vi "MotionProfiles_Control.vi"(8 "error in (no error)":errorcluster, 11 "MotionProfiles in":refnum<class "MotionProfiles.lvclass">) -> (0 "error out":errorcluster, 3 "MotionProfiles out":refnum<class "MotionProfiles.lvclass">)   [LabVIEW 2016, in "MotionProfiles.lvclass"]
uses:
  MotionProfiles.lvclass
  MotionProfiles.lvclass/MotionProfiles.ctl
  MotionProfile_InternalStateEnum.ctl
  MotionProfile_TalonSetValueEnum.ctl
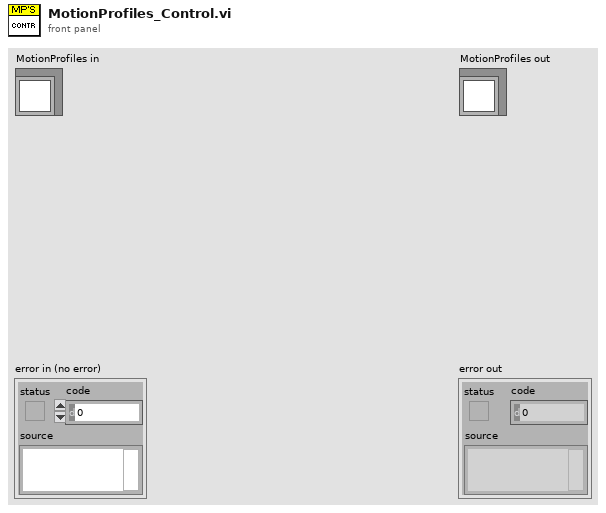
[diagram p1: front panel]
types:
  T1 = typedef "MotionProfiles.lvclass/MotionProfile_InternalStateEnum.ctl" = enum16{"Nothing", "Send Points to Talon", "Run Profile"}
  T2 = typedef "MotionProfiles.lvclass/MotionProfile_TalonSetValueEnum.ctl" = enum16{"Disable", "Enable", "Hold"}
  T3 = typedef "WPI_MotorControlDeviceRef.ctl" = cluster{"DeviceStatus":errorcluster, "Type":T4, "PWM":cluster{"PWM Channel":T5, "DeadBand":T6}, "CAN":cluster{"Device Number":u8, "SetOutput VI Ref":variant, "GetOutput VI Ref":variant, "Enable VI Ref":variant, "Disable VI Ref":variant, "Data":variant}, "Invert":bool}
  T4 = typedef "WPI_MotorControlType.ctl" = enum16{"PWM", "CAN"}
  T5 = typedef "FPGA_DIOPWMChannel.ctl" = enum8{"PWM 0", "PWM 1", "PWM 2", "PWM 3", "PWM 4", "PWM 5", "PWM 6", "PWM 7", "PWM 8", "PWM 9", "PWM MXP 0", "PWM MXP 1", "PWM MXP 2", "PWM MXP 3", "PWM MXP 4", "PWM MXP 5", "PWM MXP 6", "PWM MXP 7", "PWM MXP 8", "PWM MXP 9", "Invalid"}
  T6 = typedef "WPI_PWMDeadband.ctl" = cluster{"Name":string, "maxPositivePwm":i32, "minPositivePwm":i32, "centerPwm":i32, "maxNegativePwm":i32, "minNegativePwm":i32, "angularRange":u16}
  T7 = typedef "WPI_CANTalonSRX_GlobalStatus.ctl" = cluster{"Applied Throttle":dbl, "Module Enabled":bool, "CAN Error":errorcluster, "Closed Loop Error":dbl, "Forward Limit Switch Closed":bool, "Reverse Limit Switch Closed":bool, "Sensor Position":dbl, "Sensor Velocity":dbl, "Current":dbl, "Sticky Fault - Over Temp":bool, "Sticky Fault - Under Voltage":bool, "Sticky Fault - Forward Limit":bool, "Sticky Fault - Reverse Limit":bool, "Sticky Fault - Forward Soft Limit":bool, "Sticky Fault - Reverse Soft Limit":bool, "Brake is Enabled":bool, "Encoder Position":dbl, "Encoder Velocity":dbl, "Encoder Index Count":dbl, "Encoder A Pin State":bool, "Encoder B Pin State":bool, "Encoder Index Pin State":bool, "Analog In":dbl, "Analog In Velocity":dbl, "Temperature (C)":dbl, "Battery Voltage":dbl, "Control 5 Is Supported":bool, "Current Profile Slot Select":dbl, "Pos Div 8":bool, "Vel Div 4":bool, "Pulse Width Position":i32, "Pulse Width Velocity":i32, "Pulse Width Rise To Rise (us)":i32, "Pulse Width Rise To Fall (us)":i32, "Mot Prof Active Is Under Run":bool, "Mot Prof Active Has Under Run":bool, "Mot Prof Active Is Last":bool, "Mot Prof Active Velocity Only":bool, "Mot Prof Active Is Valid":bool, "Mot Prof Buffer Is Full":bool, "Mot Prof Active Profile Slot Select":i32, "Mot Prof NextID":i32, "Mot Prof Count":i32, "Mot Prof Active Velocity":dbl, "Mot Prof Active Position":dbl, "Mot Prof Output Enable":i32, "UsageFrame":u32, "Motion Magic Active Trajectory":cluster{"Velocity":dbl, "Position":dbl}}
  T8 = typedef "WPI_CANTalonSRX_MotionProfileTrajectoryPt.ctl" = cluster{"Duration Ms":u8, "Velocity":dbl, "Position":dbl, "Profile Slot Select":u8, "Is Last":bool, "Velocity Only":bool, "Zero Position":bool, "Compress Code":u8, "Same Velocity":i32, "Delta Position":i32, "Count":u8}
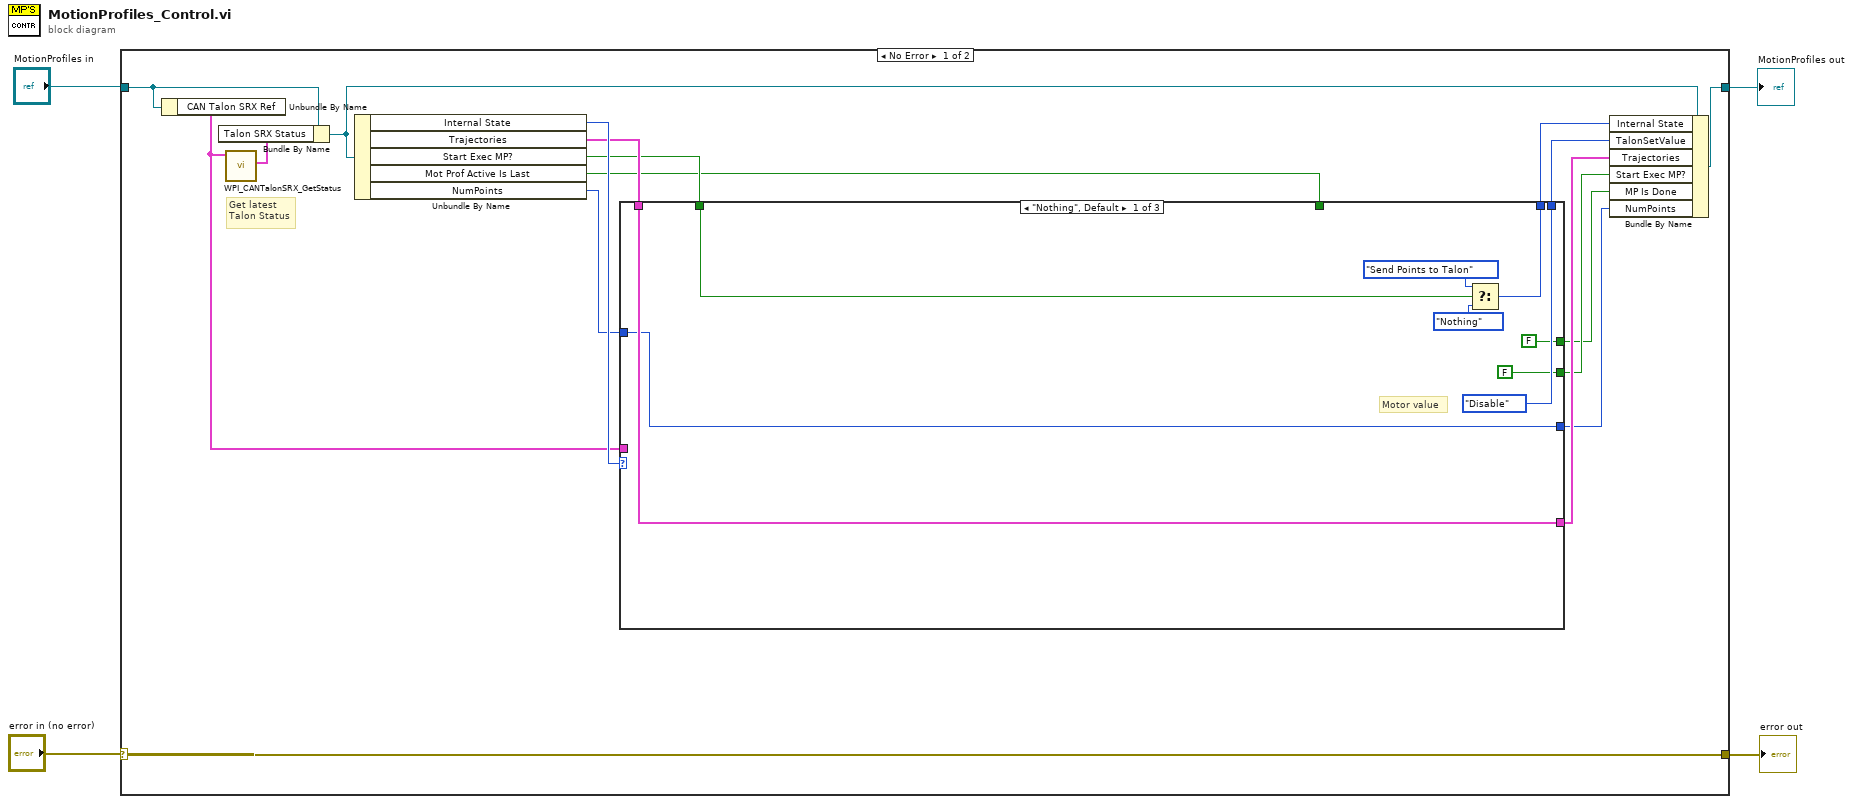
[diagram p0: block diagram]
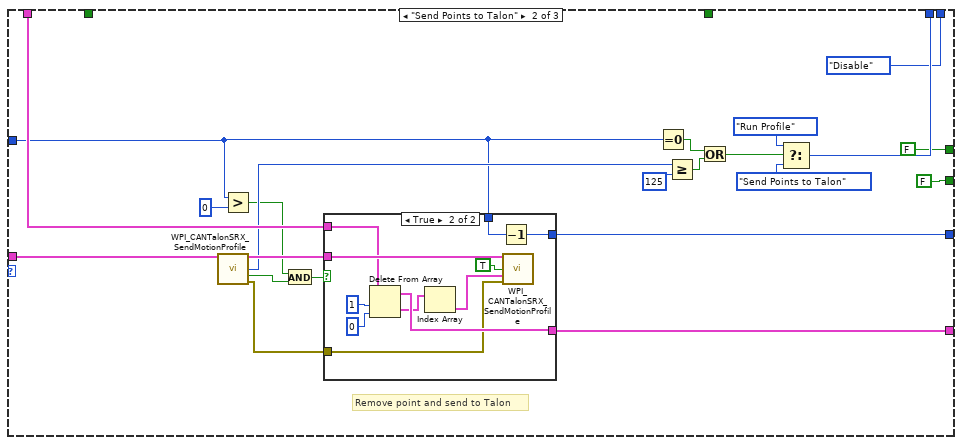
[diagram p2: hidden frame]
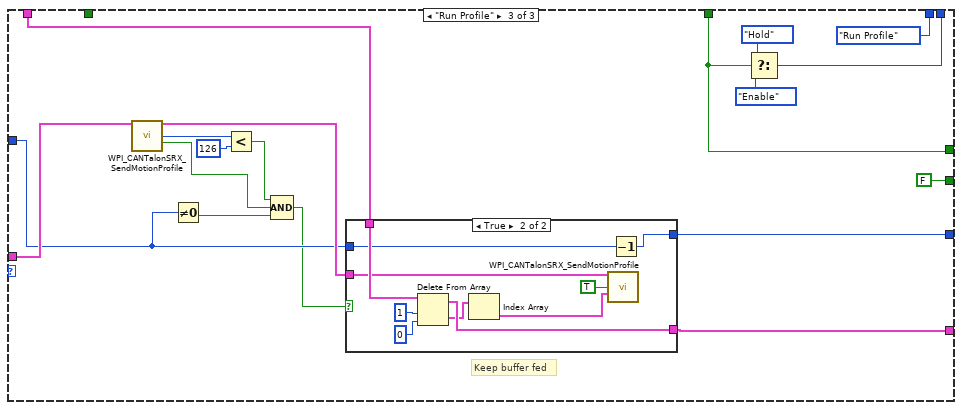
[diagram p4: hidden frame]
diagram:
  n1 = case shown="No Error" "error in (no error)" {
    selector: "error in (no error)" -> [w21 w97]
    tunnel: [w21 w97] -> w3
    tunnel: [w18 w96] -> w1
    tunnel: "MotionProfiles in" -> [w20 w96]
    frame No Error {
      # "Get latest\nTalon Status"
      n2 = Unbundle By Name(w20) -> ("CAN Talon SRX Ref"=w12:T3)
      n3 = call <vilib>:"WPI_CANTalonSRX_GetStatus.vi"("CAN Talon SRX Ref"=w12) -> ("Talon SRX Status"=w19:T7)  [unwired: 8 in, 2 out]
      n4 = Bundle By Name(cluster=w20, "Talon SRX Status"=w19) -> (w17:refnum<class "MotionProfiles.lvclass">)
      n5 = Unbundle By Name(w17) -> ("Internal State"=w14:T1, "Trajectories"=w13:T8[], "Start Exec MP?"=w10:bool, "Mot Prof Active Is Last"=w8:bool, "NumPoints"=w7:u16)
      n6 = case shown="\"Nothing\", Default" w14 {
        tunnel: [w28 w47 MotionProfile_InternalStateEnum."Run Profile" ("Internal State")] -> w16
        tunnel: [MotionProfile_TalonSetValueEnum."Disable" ("TalonSetValue") MotionProfile_TalonSetValueEnum."Disable" ("TalonSetValue") w76] -> w15
        tunnel: w13 -> [w24 w46 w81]
        tunnel: w12 -> [_ w45 w80]
        tunnel: [w24 w44 w79] -> w11
        tunnel: w10 -> [w26 _ _]
        tunnel: [FALSE ("Start Exec MP?") FALSE ("Start Exec MP?") FALSE] -> w9
        tunnel: w8 -> [_ _ w72]
        tunnel: w7 -> [w22 w32 w70]
        tunnel: [FALSE ("Mot Prof Active Is Last") FALSE ("Mot Prof Active Is Last") w72] -> w6
        tunnel: [w22 w31 w71] -> w5
        frame "Nothing", Default {
          # "Motor value"
          n7 = Select(t=MotionProfile_InternalStateEnum."Send Points to Talon" ("Internal State"), s=w26, f=MotionProfile_InternalStateEnum."Nothing" ("Internal State")) -> (s? t:f=w28:T1)
        }
        frame "Send Points to Talon" {
          # "Remove point and send to Talon"
          n8 = call <vilib>:"WPI_CANTalonSRX_SendMotionProfile.vi"("CAN Talon SRX Ref"=w45) -> ("CAN Talon SRX Ref Out"=w52:T3, "Count"=w42:u32, "Ready For Next"=w35:bool, "error out"=w51:errorcluster)  [unwired: 11 in]
          n9 = Greater?(x=w32, y=u16 0) -> (0:w34:bool)
          n10 = And(x=w34, y=w35) -> (x .and. y?=w36:bool)
          n11 = case shown="True" w36 {
            tunnel: w52 -> [_ w64]
            tunnel: [w54 w63] -> w44
            tunnel: w51 -> [_ w60]
            tunnel: w46 -> [w54 w59]
            tunnel: w32 -> [w53 w56]
            tunnel: [w53 w55] -> w31
            frame False {
            }
            frame True {
              n12 = Delete From Array(array=w59, length=1, index=0) -> (deleted portion=w58:T8[], array with subset deleted=w63:T8[])
              n13 = Index Array(array=w58) -> (element=w57:T8)  [unwired: 1 in]
              n14 = Decrement(x=w56) -> (x-1=w55:u16)
              n15 = call <vilib>:"WPI_CANTalonSRX_SendMotionProfile.vi"("CAN Talon SRX Ref"=w64, "Push"=TRUE, "New Point"=w57, "error in"=w60) -> ()  [unwired: 8 in, 4 out]
            }
          }
          n16 = Equal To 0?(x=w32) -> (x = 0?=w33:bool)
          n17 = Greater Or Equal?(x=w42, y=u32 125) -> (x >= y?=w41:bool)
          n18 = Or(x=w33, y=w41) -> (x .or. y?=w40:bool)
          n19 = Select(t=MotionProfile_InternalStateEnum."Run Profile" ("Internal State"), s=w40, f=MotionProfile_InternalStateEnum."Send Points to Talon" ("Internal State")) -> (s? t:f=w47:T1)
        }
        frame "Run Profile" {
          # "Keep buffer fed"
          n20 = call <vilib>:"WPI_CANTalonSRX_SendMotionProfile.vi"("CAN Talon SRX Ref"=w80) -> ("CAN Talon SRX Ref Out"=w78:T3, "Count"=w83:u32, "Ready For Next"=w67:bool)  [unwired: 11 in, 1 out]
          n21 = Not Equal To 0?(x=w70) -> (x != 0?=w66:bool)
          n22 = Less?(x=w83, y=u32 126) -> (x < y?=w68:bool)
          n23 = Compound Arithmetic op=AND(w68, w67, w66) -> (w69:bool)
          n24 = case shown="True" w69 {
            tunnel: [w85 w94] -> w79
            tunnel: w81 -> [w85 w91]
            tunnel: w78 -> [_ w88]
            tunnel: w70 -> [w84 w87]
            tunnel: [w84 w86] -> w71
            frame False {
            }
            frame True {
              n25 = Delete From Array(array=w91, length=1, index=0) -> (deleted portion=w90:T8[], array with subset deleted=w94:T8[])
              n26 = Index Array(array=w90) -> (element=w89:T8)  [unwired: 1 in]
              n27 = call <vilib>:"WPI_CANTalonSRX_SendMotionProfile.vi"("CAN Talon SRX Ref"=w88, "Push"=TRUE, "New Point"=w89) -> ()  [unwired: 9 in, 4 out]
              n28 = Decrement(x=w87) -> (x-1=w86:u16)
            }
          }
          n29 = Select(t=MotionProfile_TalonSetValueEnum."Hold" ("TalonSetValue"), s=w72, f=MotionProfile_TalonSetValueEnum."Enable" ("TalonSetValue")) -> (s? t:f=w76:T2)
        }
      }
      n30 = Bundle By Name(cluster=w17, "Internal State"=w16, "TalonSetValue"=w15, "Trajectories"=w11, "Start Exec MP?"=w9, "MP Is Done"=w6, "NumPoints"=w5) -> (w18:refnum<class "MotionProfiles.lvclass">)
    }
    frame Error {
    }
  }
  "error out" <- w3
  "MotionProfiles out" <- w1
